vi "SVL Limit Testing (scalar).vi"(8 "error in (no error)":errorcluster, 9 "lower limit":dbl=-inf format="%.2f", 10 "upper limit":dbl=inf format="%.2f", 11 "value in":dbl format="%.2f") -> (0 "error out":errorcluster, 1 "output values":T1(graph), 3 "test passed?":bool)   [LabVIEW 2017, in "SoundVib_LimitTest.lvlib"]
doc: "Performs limit testing on waveforms, spectra, XY data, identified peaks, or scalar measurements. You can specify an upper and lower boundary of the envelope to define a pass range. This VI uses the defined pass range to test the input signal. VI outputs apply only to the current input signal. You can wire output values to a graph to view the limits, signal, and failures. Wire data to the<B> signal in</B> input to determine the polymorphic instance to use or manually select the instance."
uses:
  <vilib>/addons/Sound and Vibration/svt_Limit Test/SoundVib_LimitTest.lvlib
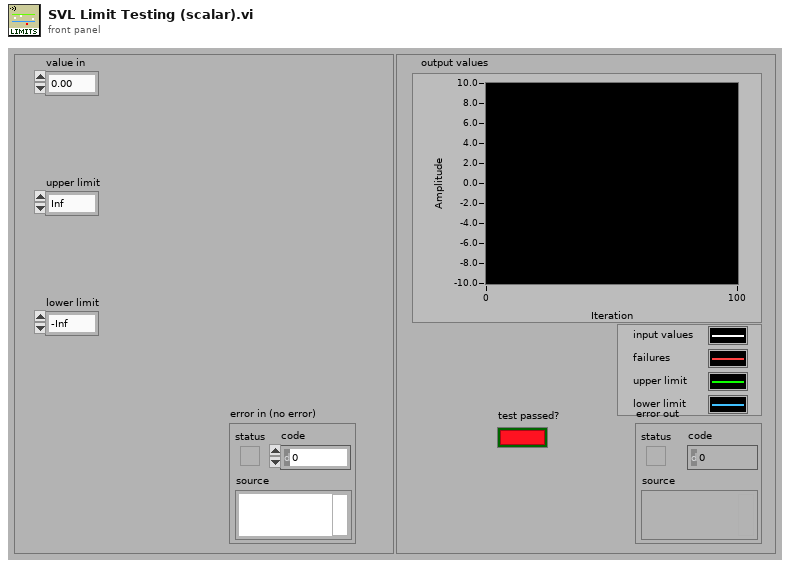
[diagram p1: front panel]
types:
  T1 = cluster{"value in":dbl, dbl, "upper limit":dbl, "lower limit":dbl}
  T2 = cluster{"value in":dbl, "failure":dbl, "upper limit":dbl, "lower limit":dbl}
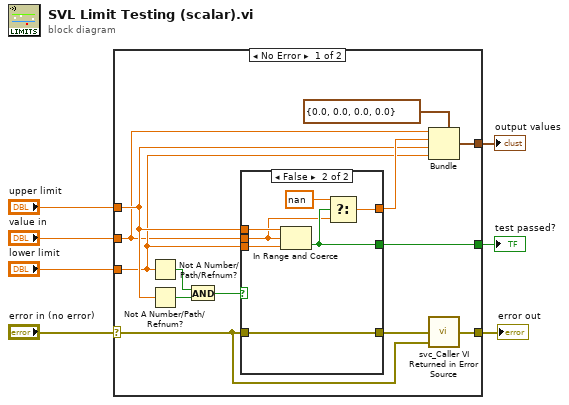
[diagram p0: block diagram]
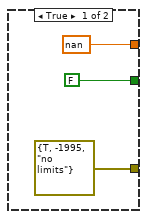
[diagram p2: hidden frame]
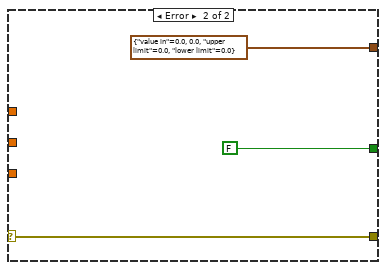
[diagram p3: hidden frame]
diagram:
  n1 = case shown="No Error" "error in (no error)" {
    selector: "error in (no error)" -> [w8 w33]
    tunnel: [w20 w33] -> w6
    tunnel: "upper limit" -> [w14 _]
    tunnel: "value in" -> [w10 _]
    tunnel: "lower limit" -> [w13 _]
    tunnel: [w18 T1 {"value in"=0.0, 0.0, "upper limit"=0.0, "lower limit"=0.0}] -> w2
    tunnel: [w17 FALSE ("lo <= x <=  hi?")] -> w1
    frame No Error {
      n2 = Not A Number/Path/Refnum?(number/path/refnum=w13) -> (NaN/Path/Refnum?=w11:bool)
      n3 = Not A Number/Path/Refnum?(number/path/refnum=w14) -> (NaN/Path/Refnum?=w15:bool)
      n4 = And(x=w11, y=w15) -> (x .and. y?=w9:bool)
      n5 = case shown="False" w9 {
        tunnel: [nan ("t") w30] -> w19
        tunnel: [FALSE w29] -> w17
        tunnel: [errorcluster {"status"=TRUE, "code"=-1995, "source"="no limits"} ("error in (no error)") w27] -> w16
        tunnel: w8 -> [_ w27]
        tunnel: w14 -> [_ w26]
        tunnel: w13 -> [_ w25]
        tunnel: w10 -> [_ w24]
        frame True {
        }
        frame False {
          n6 = In Range and Coerce(upper limit=w26, x=w24, lower limit=w25) -> (In Range?=w29:bool)  [unwired: 1 out]
          n7 = Select(t=nan, s=w29, f=w24) -> (s? t:f=w30:dbl)
        }
      }
      n8 = Bundle(cluster=T2 {"value in"=0.0, "failure"=0.0, "upper limit"=0.0, "lower limit"=0.0} ("output values"), "value in"=w10, "failure"=w19, "upper limit"=w14, "lower limit"=w13) -> (w18:T2)
      n9 = call <vilib>:"svc_Caller VI Returned in Error Source.vi"("warning input to caller"=w8, "error in (no error)"=w16) -> ("error out"=w20:errorcluster)  [unwired: 3 in]
    }
    frame Error {
    }
  }
  "error out" <- w6
  "output values" <- w2
  "test passed?" <- w1
